vi "Read Colors.vi"(9 "Decoration in":refnum<class "Decoration.lvclass">) -> (3 "Decoration out":refnum<class "Decoration.lvclass">, 4 "Colors":T1)   [LabVIEW 2014, in "Raspberry Pi Compatible Compiler for LabVIEW.lvlib" / "Decoration.lvclass"]
uses:
  Decoration.lvclass
  <vilib>/Utility/miscctls.llb/LVForegroundBackgroundColorsTypeDef.ctl
  Decoration.lvclass/Decoration.ctl
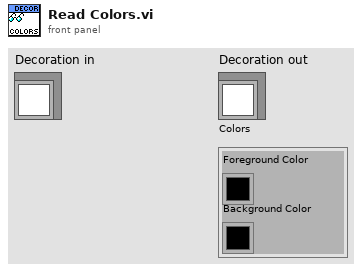
[diagram p1: front panel]
types:
  T1 = typedef "LVForegroundBackgroundColorsTypeDef.ctl" = cluster{"Foreground Color":u32, "Background Color":u32}
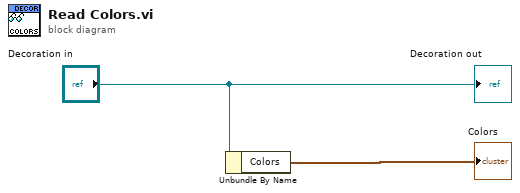
[diagram p0: block diagram]
diagram:
  n1 = Unbundle By Name("Decoration in") -> ("Colors"=→"Colors":T1)
  "Decoration out" <- "Decoration in"
